vi "test Add Multiple Custom Devices.vi"(8 "error in":errorcluster, 11 "TestCase in":refnum<class "Scripting.lvclass">) -> (0 "error out":errorcluster, 3 "TestCase out":refnum<class "Scripting.lvclass">)   [LabVIEW 2020, in "Scripting.lvclass"]
uses:
  Scripting.lvclass
  <vilib>/addons/_JKI Toolkits/VI Tester/TestCase.llb/TestCase.lvclass
  Scripting/Ballard MIL-STD-1553 Scripting.lvlib
  C:/Program Files (x86)/National Instruments/LabVIEW 2020/vi.lib/addons/_JKI Toolkits/VI Tester/TestCase.llb/TestCase.lvclass
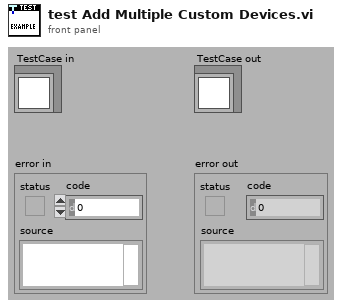
[diagram p1: front panel]
types:
  T1 = typedef "Custom Device API.lvlib/Custom Device Item Ref.ctl" = u64
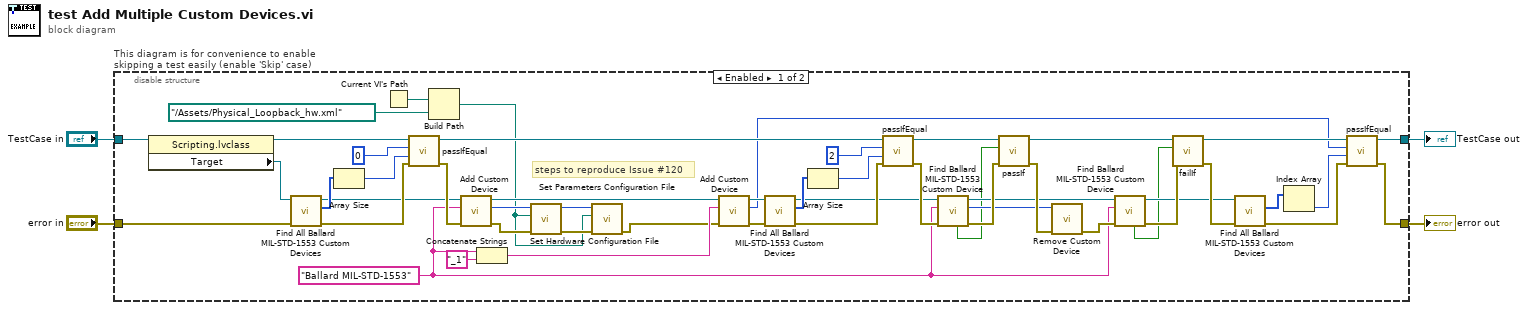
[diagram p0: block diagram]
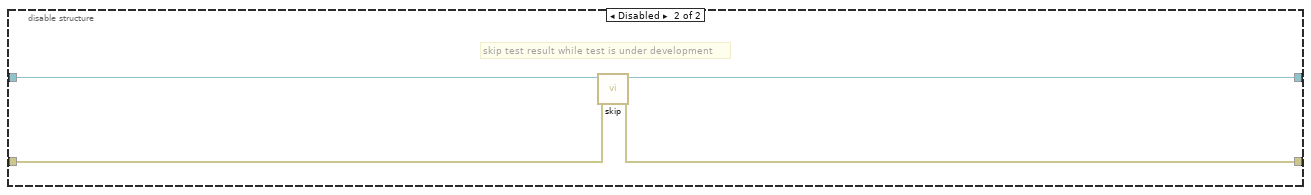
[diagram p2: hidden frame]
diagram:
  n1 = disable-structure "This diagram is for convenience to enable skipping a test easily (enable 'Skip' case)" shown="Enabled" {
    disable-tunnel: "TestCase in" -> [w21 w58]
    disable-tunnel: [w23 w56] -> w1
    disable-tunnel: [w22 w57] -> w3
    disable-tunnel: "error in" -> [w54 w55]
    frame Enabled {
      w31 = "Ballard MIL-STD-1553" ("name")
      # "steps to reproduce Issue #120"
      n2 = property class="Scripting.lvclass"(reference=w21) -> (reference out=w19:refnum<class "Scripting.lvclass">, "Target"=w20:refnum<k24>)  [unwired: 1 in, 1 out]
      n3 = call "Find All Ballard MIL-STD-1553 Custom Devices.vi"("error in"=w54, "target in"=w20) -> ("error out"=w50:errorcluster, "Ballard MIL-STD-1553 custom devices"=w53:T1[], "target out"=w48:refnum<k24>)  [unwired: 7 in]
      n4 = Array Size(array=w53) -> (size(s)=w52:i32)
      n5 = Current VI's Path() -> (path=w15:path)
      n6 = call-dynamic "passIfEqual.vi"("error in (no error)"=w50, "y"=w52, "x"=0 ("size(s)"), "TestCase in"=w19) -> ("error out"=w49:errorcluster, "TestCase out"=w18:refnum<class "Scripting.lvclass">)  [unwired: 6 in]
      n7 = Build Path(base path=w15, name or relative path=path "../Assets/Physical_Loopback_hw.xml") -> (appended path=w10:path)
      n8 = call "Add Custom Device.vi"("error in"=w49, "name"=w31, "target in"=w48) -> ("error out"=w16:errorcluster, "Ballard MIL-STD 1553 custom device"=w17:T1, "target out"=w46:refnum<k24>)  [unwired: 6 in]
      n9 = Concatenate Strings(w31, "_1" ("string")) -> (w45:string)
      n10 = call "Set Hardware Configuration File.vi"("error in"=w16, "hardware configuration file path"=w10, "Ballard MIL-STD 1553 custom device in"=w17) -> ("error out"=w12:errorcluster, "Ballard MIL-STD 1553 custom device out"=w13:T1)  [unwired: 7 in]
      n11 = call "Set Parameters Configuration File.vi"("error in"=w12, "parameters configuration file path"=w10, "Ballard MIL-STD 1553 custom device in"=w13) -> ("error out"=w11:errorcluster)  [unwired: 7 in, 1 out]
      n12 = call "Add Custom Device.vi"("error in"=w11, "name"=w45, "target in"=w46) -> ("error out"=w44:errorcluster, "Ballard MIL-STD 1553 custom device"=w5:T1, "target out"=w43:refnum<k24>)  [unwired: 6 in]
      n13 = call "Find All Ballard MIL-STD-1553 Custom Devices.vi"("error in"=w44, "target in"=w43) -> ("error out"=w39:errorcluster, "Ballard MIL-STD-1553 custom devices"=w40:T1[], "target out"=w37:refnum<k24>)  [unwired: 7 in]
      n14 = Array Size(array=w40) -> (size(s)=w41:i32)
      n15 = call-dynamic "passIfEqual.vi"("error in (no error)"=w39, "y"=w41, "x"=2 ("size(s)"), "TestCase in"=w18) -> ("error out"=w38:errorcluster, "TestCase out"=w36:refnum<class "Scripting.lvclass">)  [unwired: 6 in]
      n16 = call "Find Ballard MIL-STD-1553 Custom Device.vi"("error in"=w38, "name"=w31, "target in"=w37) -> ("error out"=w35:errorcluster, "Ballard MIL-STD 1553 custom device"=w33:T1, "target out"=w30:refnum<k24>, "found?"=w9:bool)  [unwired: 5 in]
      n17 = call-dynamic "passIf.vi"("error in (no error)"=w35, "pass"=w9, "TestCase in"=w36) -> ("error out"=w34:errorcluster, "TestCase out"=w29:refnum<class "Scripting.lvclass">)  [unwired: 7 in]
      n18 = call "Remove Custom Device.vi"("error in"=w34, "Ballard MIL-STD 1553 custom device"=w33) -> ("error out"=w32:errorcluster)  [unwired: 9 in]
      n19 = call "Find Ballard MIL-STD-1553 Custom Device.vi"("error in"=w32, "name"=w31, "target in"=w30) -> ("error out"=w28:errorcluster, "target out"=w26:refnum<k24>, "found?"=w8:bool)  [unwired: 5 in, 1 out]
      n20 = call-dynamic "failIf.vi"("error in (no error)"=w28, "fail"=w8, "TestCase in"=w29) -> ("error out"=w27:errorcluster, "TestCase out"=w25:refnum<class "Scripting.lvclass">)  [unwired: 7 in]
      n21 = call "Find All Ballard MIL-STD-1553 Custom Devices.vi"("error in"=w27, "target in"=w26) -> ("error out"=w24:errorcluster, "Ballard MIL-STD-1553 custom devices"=w7:T1[])  [unwired: 7 in, 1 out]
      n22 = Index Array(array=w7) -> (element=w6:T1)  [unwired: 1 in]
      n23 = call-dynamic "passIfEqual.vi"("error in (no error)"=w24, "y"=w6, "x"=w5, "TestCase in"=w25) -> ("error out"=w22:errorcluster, "TestCase out"=w23:refnum<class "Scripting.lvclass">)  [unwired: 6 in]
    }
    frame Disabled {
      # "skip test result while test is under development"
      n24 = call <vilib>:"skip.vi"("error in (no error)"=w55, "TestCase in"=w58) -> ("error out"=w57:errorcluster, "TestCase out"=w56:refnum<class "Scripting.lvclass">)  [unwired: 8 in]
    }
  }
  "error out" <- w3
  "TestCase out" <- w1
